vi "ZScan_XYZCompute.vi"(11 "Reference Data":T1={"Refrence data path"=path "", "Reference Rectangle"=[], "AOL Z"=0.0, "No of pixels in a miniscan "=[], "Threshold"=[], "No of miniscans"=[], "Full Frame Size"=0, "Reference Image"=refnum, "dwelltime"=0.0, "Zoom"=0.0, "Field of View"=0.0, "Z Step"=1, "Z pixels"=1, "Z Lines"=1, "Z Ignore"=1, "Laser"=1, "Auto centering"=FALSE}) -> (1 "XYZ Stop":cluster{"X":dbl, "Y":dbl, "Z":dbl}[](array[cluster]), 3 "XYZ Start":cluster{"X":dbl, "Y":dbl, "Z":dbl}[](array[cluster]))   [LabVIEW 2020]
uses:
  Typedefs/Reference_Globals.ctl
  <vilib>/vision/Image Controls.llb/IMAQ Image.ctl
panel:
  in  "y":dbl=1.14
  out "Zoom":dbl
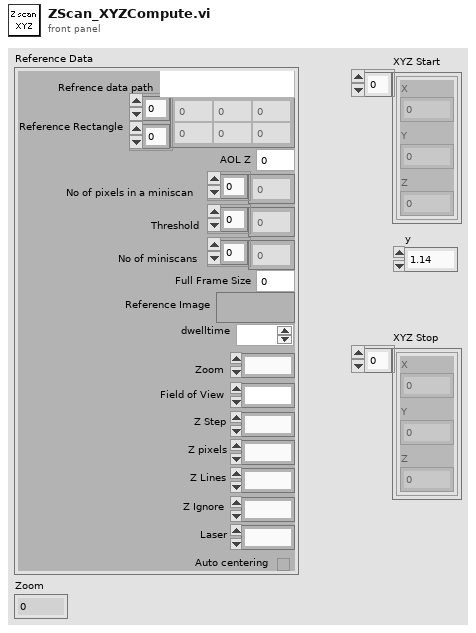
[diagram p1: front panel]
types:
  T1 = typedef "Reference_Globals.ctl" = cluster{"Refrence data path":path, "Reference Rectangle":i16[][], "AOL Z":dbl, "No of pixels in a miniscan ":i32[], "Threshold":i16[], "No of miniscans":i32[], "Full Frame Size":u16, "Reference Image":T2, "dwelltime":dbl, "Zoom":dbl, "Field of View":dbl, "Z Step":i8, "Z pixels":i32, "Z Lines":u8, "Z Ignore":u8, "Laser":u8, "Auto centering":bool}
  T2 = typedef "IMAQ Image.ctl" = refnum<image>
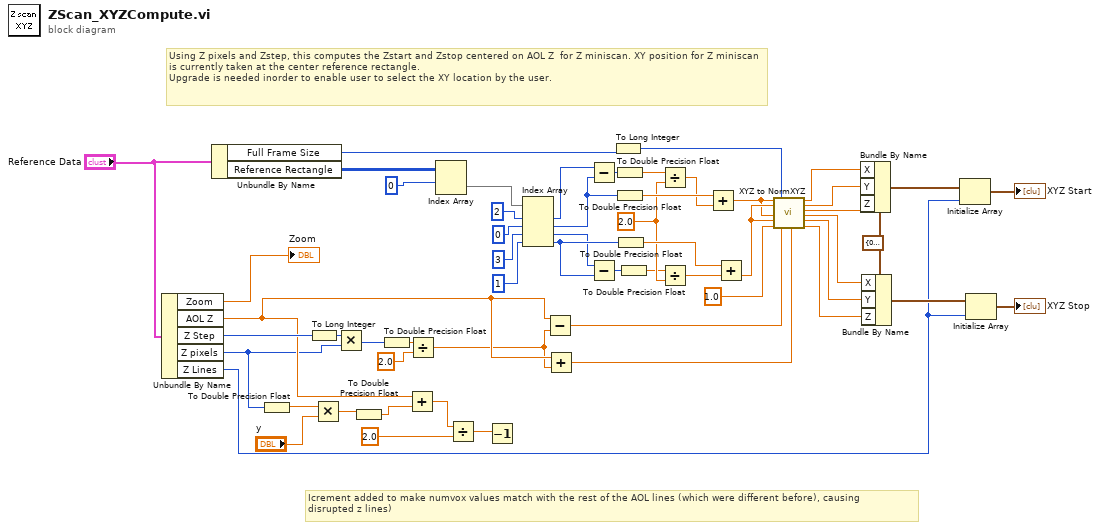
[diagram p0: block diagram]
diagram:
  w50 = cluster{"X":dbl, "Y":dbl, "Z":dbl} {"X"=0.0, "Y"=0.0, "Z"=0.0} ("XYZ")
  w38 = 2.0
  # "Icrement added to make numvox values match with the rest of the AOL lines (which were different before), causing \ndisrupted z lines)"
  # "Using Z pixels and Zstep, this computes the Zstart and Zstop centered on AOL Z  for Z miniscan. XY position for Z miniscan is currently taken at the center reference rectangle.\nUpgrade is needed inorder to enable user to select the XY location by the user."
  n1 = Unbundle By Name("Reference Data") -> ("Zoom"=→"Zoom":dbl, "AOL Z"=w10:dbl, "Z Step"=w24:i8, "Z pixels"=w2:i32, "Z Lines"=w21:u8)
  n2 = Unbundle By Name("Reference Data") -> ("Full Frame Size"=w47:u16, "Reference Rectangle"=w25:i16[][])
  n3 = To Double Precision Float(number=w2) -> (double precision float=w3:dbl)
  n4 = To Long Integer(number=w24) -> (32bit integer=w4:i32)
  n5 = Multiply(x=w3, y="y") -> (x*y=w12:dbl)
  n6 = Multiply(x=w4, y=w2) -> (x*y=w5:i32)
  n7 = To Double Precision Float(number=w12) -> (double precision float=w9:dbl)
  n8 = To Double Precision Float(number=w5) -> (double precision float=w6:dbl)
  n9 = Add(x=w10, y=w9) -> (x+y=w11:dbl)
  n10 = Divide(x=w6, y=2.0) -> (x/y=w1:dbl)
  n11 = Index Array(array=w25, index (row)=0) -> (element=w27:i16[])  [unwired: 1 in]
  n12 = Divide(x=w11, y=2.0) -> (x/y=w8:dbl)
  n13 = Decrement(x=w8) -> ()  [unwired: 1 out]
  n14 = Index Array(array=w27, index #1=2 ("index"), index #2=0 ("index"), index #3=3 ("index"), index #4=1 ("index")) -> (element #1=w32:i16, element #2=w40:i16, element #3=w33:i16, element #4=w42:i16)
  n15 = Subtract(x=w10, y=w1) -> (x-y=w16:dbl)
  n16 = Add(x=w10, y=w1) -> (x+y=w15:dbl)
  n17 = Subtract(x=w32, y=w40) -> (x-y=w34:i16)
  n18 = Subtract(x=w33, y=w42) -> (x-y=w35:i16)
  n19 = To Long Integer(number=w47) -> (32bit integer=w48:i32)
  n20 = To Double Precision Float(number=w34) -> (double precision float=w37:dbl)
  n21 = To Double Precision Float(number=w40) -> (double precision float=w44:dbl)
  n22 = To Double Precision Float(number=w42) -> (double precision float=w43:dbl)
  n23 = To Double Precision Float(number=w35) -> (double precision float=w36:dbl)
  n24 = Divide(x=w37, y=w38) -> (x/y=w39:dbl)
  n25 = Divide(x=w36, y=w38) -> (x/y=w41:dbl)
  n26 = Add(x=w44, y=w39) -> (x+y=w45:dbl)
  n27 = Add(x=w43, y=w41) -> (x+y=w46:dbl)
  n28 = call "XYZ to NormXYZ.vi"("X start"=w45, "Y start"=w46, "X stop"=w45, "Y stop"=w46, "Zoom (either ref or main zoom)"=1.0, "FrameSize"=w48, "Z start"=w16, "Z stop"=w15) -> ("Norm X Start"=w51:dbl, "Norm Y Start"=w52:dbl, "Norm Z Start"=w53:dbl, "Norm X Stop"=w54:dbl, "Norm Y Stop"=w55:dbl, "Norm Z Stop"=w56:dbl)  [unwired: 6 in]
  n29 = Bundle By Name(cluster=w50, "X"=w51, "Y"=w52, "Z"=w53) -> (w23:cluster{"X":dbl, "Y":dbl, "Z":dbl})
  n30 = Bundle By Name(cluster=w50, "X"=w54, "Y"=w55, "Z"=w56) -> (w22:cluster{"X":dbl, "Y":dbl, "Z":dbl})
  n31 = Initialize Array(w23, w21) -> (→"XYZ Start":cluster{"X":dbl, "Y":dbl, "Z":dbl}[])
  n32 = Initialize Array(w22, w21) -> (→"XYZ Stop":cluster{"X":dbl, "Y":dbl, "Z":dbl}[])
